vi "Stop Module.vi"(8 "error in (no error)":errorcluster, 9 "Wait for Module to stop? (F)":bool, 10 "Origin":string, 11 "Module ID":i32=-1) -> (0 "error out":errorcluster)   [LabVIEW 2024, in "Thermal Chamber.lvlib"]
doc: "Send the Stop request to the Module's Main.vi. If <b>Wait for Module to stop?</b> is TRUE, then this VI will not complete execution until the Module Main VI has stopped running.\n\n<b>Note:</b> If the cloneable module is running as singleton, then the 'Wait for Module to stop?' input is ignored... this VI will <b>always</b> wait until a cloneable Main VI running as singleton has stopped running.\n_____\nBased on DQMH Project Template 6.0.0.91.\n\n<b>Note:</b> This VI was modified by the <b>Validate DQMH Module</b> tool to upgrade it to the DQMH 5.0 approach to destroying cloneable module event references.\n\n<b>Note:</b> This VI was modified by the <b>Validate DQMH Module</b> tool to remove the Status Updated.vi subVI call."
uses:
  Thermal Chamber.lvlib
  Stop Argument--cluster.ctl
  Module Running State--enum.ctl
  Main.vi
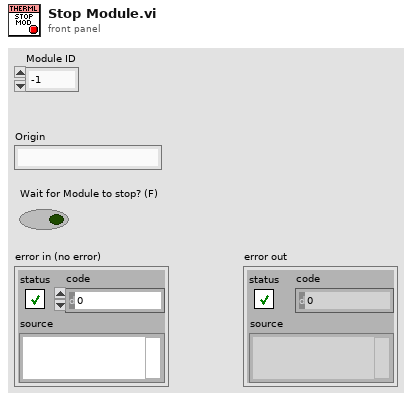
[diagram p1: front panel]
types:
  T1 = typedef "Thermal Chamber.lvlib/Module Running State--enum.ctl" = enum16{"Not Running", "Running as Cloneable", "Running as Singleton"}
  T2 = typedef "Thermal Chamber.lvlib/Stop Argument--cluster.ctl" = cluster{"Module ID":i32, "Origin":string, "Exit via Stop Module Req?":bool, "Wait for Module to stop?":bool}
  T3 = typedef "Thermal Chamber.lvlib/Request Events--cluster.ctl" = cluster{"Stop Module":refnum<user-event>, "Show Panel":refnum<user-event>, "Hide Panel":refnum<user-event>, "Show Diagram":refnum<user-event>, "Get Module Execution Status":refnum<user-event>, "Initialize":refnum<user-event>, "Shutdown":refnum<user-event>, "Set Temp Setpoint":refnum<user-event>, "Set Temp Ramp Rate":refnum<user-event>, "Set Temp Control State":refnum<user-event>, "Get Temp Feedback":refnum<user-event>, "Read Controller Data":refnum<user-event>}
  T4 = enum32{"Bad", "Idle", "Run top level", "Running"}
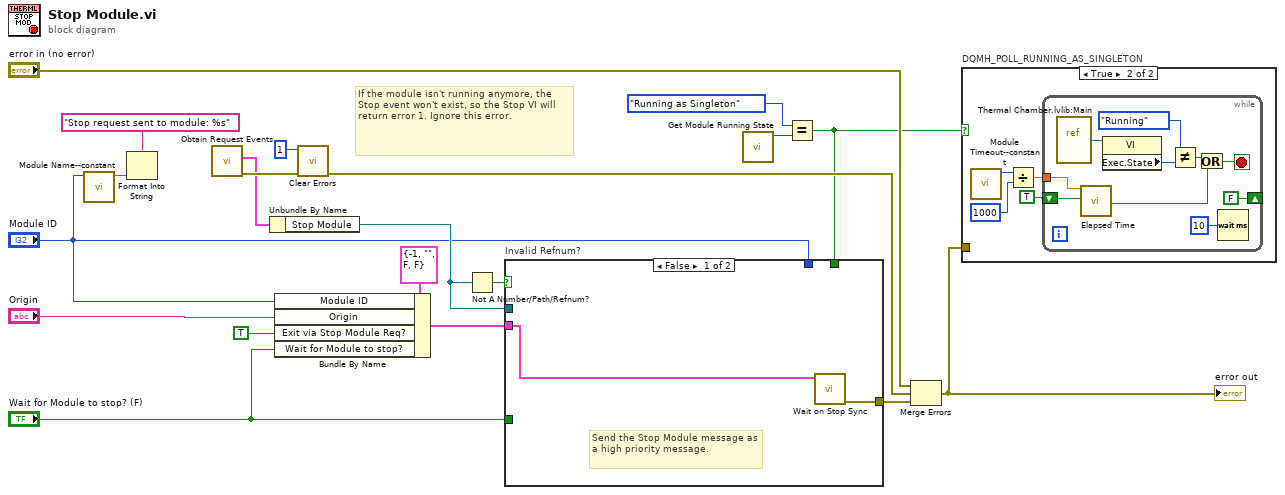
[diagram p0: block diagram]
diagram:
  # "If the module isn't running anymore, the Stop event won't exist, so the Stop VI will return error 1. Ignore this error."
  n1 = call "Module Name--constant.vi"("Module ID"="Module ID") -> ("Module Name"=w18:string)  [unwired: 10 in]
  n2 = Format Into String(format string="Stop request sent to module: %s", w18) -> ()  [unwired: 2 in, 2 out]
  n3 = call "Obtain Request Events.vi"() -> ("error out"=w12:errorcluster, "Thermal Chamber Request Events"=w10:T3)  [unwired: 10 in]
  n4 = Unbundle By Name(w10) -> ("Stop Module"=w14:refnum<user-event>)
  n5 = Bundle By Name(cluster=T2 {"Module ID"=-1, "Origin"="", "Exit via Stop Module Req?"=FALSE, "Wait for Module to stop?"=FALSE} ("event data"), "Module ID"="Module ID", "Origin"="Origin", "Exit via Stop Module Req?"=TRUE, "Wait for Module to stop?"="Wait for Module to stop? (F)") -> (w13:T2)
  n6 = call <vilib>:"Clear Errors.vi"("error in (no error)"=w12, "specific error code to clear (0: all)"=1) -> ("error out"=w9:errorcluster)  [unwired: 4 in, 1 out]
  n7 = Not A Number/Path/Refnum?(number/path/refnum=w14) -> (NaN/Path/Refnum?=w15:bool)
  n8 = call "Get Module Running State.vi"() -> ("Module Running State"=w4:T1)  [unwired: 11 in]
  n9 = Equal?(x=Module_Running_State--enum."Running as Singleton", y=w4) -> (x = y?=w3:bool)
  n10 = case "Invalid Refnum?" shown="False" w15 {
    tunnel: [w21 _] -> w8
    tunnel: w13 -> [w22 _]
    tunnel: w14 -> [_ _]
    tunnel: "Module ID" -> [_ _]
    tunnel: "Wait for Module to stop? (F)" -> [_ _]
    tunnel: w3 -> [_ _]
    frame False {
      # "Send the Stop Module message as a high priority message."
      n11 = call "Wait on Stop Sync.vi"("Stop Argument"=w22) -> ("error out"=w21:errorcluster)  [unwired: 10 in]
    }
    frame True {
      # "Module is exiting. No need to send the standard \"not running\" error that is sent in other request VIs."
    }
  }
  n12 = Merge Errors("error in (no error)", w9, w8) -> (w1:errorcluster)
  "error out" <- w1
  n13 = case "DQMH_POLL_RUNNING_AS_SINGLETON" shown="True" w3 {
    tunnel: w1 -> [_ _]
    frame False {
    }
    frame True {
      n14 = call "Module Timeout--constant.vi"() -> ("Module Timeout"=w26:i32)  [unwired: 11 in]
      n15 = Divide(x=w26, y=1000) -> (x/y=w24:dbl)
      n16 = while {
        tunnel: w24 -> [w29]
        shift-right: [FALSE] -> _
        shift-left: TRUE -> [w30]
        stop <- w32 stop-if-true
        n17 = vi-ref "Thermal Chamber.lvlib:Main.vi"() -> (w36:refnum<vi>)
        n18 = call "Elapsed Time"("Time Target (s)"=w29, "Reset"=w30) -> ("Time has Elapsed"=w28:bool)  [unwired: 10 in, 7 out]
        n19 = property class="VI"(reference=w36) -> ("Exec.State"=w35:T4)  [unwired: 1 in, 2 out]
        n20 = Not Equal?(x=T4."Running", y=w35) -> (x != y?=w33:bool)
        n21 = Or(x=w33, y=w28) -> (x .or. y?=w32:bool)
        n22 = Wait (ms)(milliseconds to wait=u32 10) -> ()  [unwired: 1 out]
      }
    }
  }
